vi "Test Executive.vi"() -> ()   [LabVIEW 2020]
uses:
  Library - Test Executive.llb/Test Executive - Globals.vi
  Library - Test Executive.llb/Test Executive.lvlib
panel:
  in  "Tab Control":T1(tab)
  in  "Serial Number":string
  out "Sequence":string
  out "Report Text":string
  in  "Operator":string
  in  "Save Report":bool
  in  "Clear Report Text":bool
  out "Sequence Name":string="None"
  in  "Abort Button":bool
  in  "Sequence Run":bool
  in  "Sequence Load":bool
  in  "Results Analyser":bool
  in  "Power Down":bool
  in  "Power Up":bool
  in  "Test":u16(ring) items=["1 Current Consumption", "2 Firmware Revision", "3 Indicators", "4 Gain", "5 Sensitivity"]
  in  "Check Test Equipment":bool
  out "errors":errorcluster
  in  "Power Down":bool
  in  "Power Up":bool
  in  "Reset All":bool
  in  "Run Single Test":bool
  out "Help Text":string="This is some help text\n"
  out "Abort":bool
  out "Error":bool
  out "Running":bool
  in  "Quit":bool
  # "Sequence"
  # "Progress"
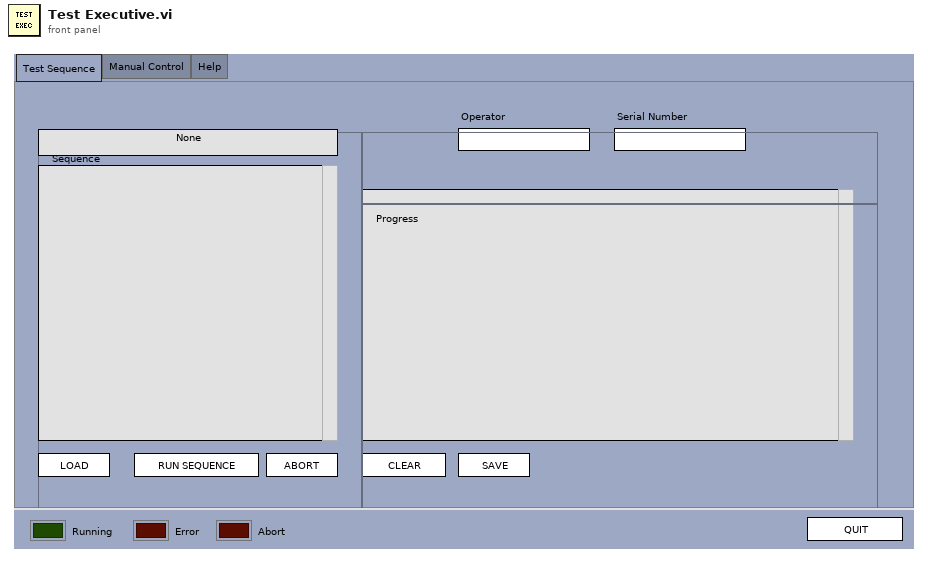
[diagram p1: front panel]
types:
  T1 = enum32{"Test Sequence", "Manual Control", "Help"}
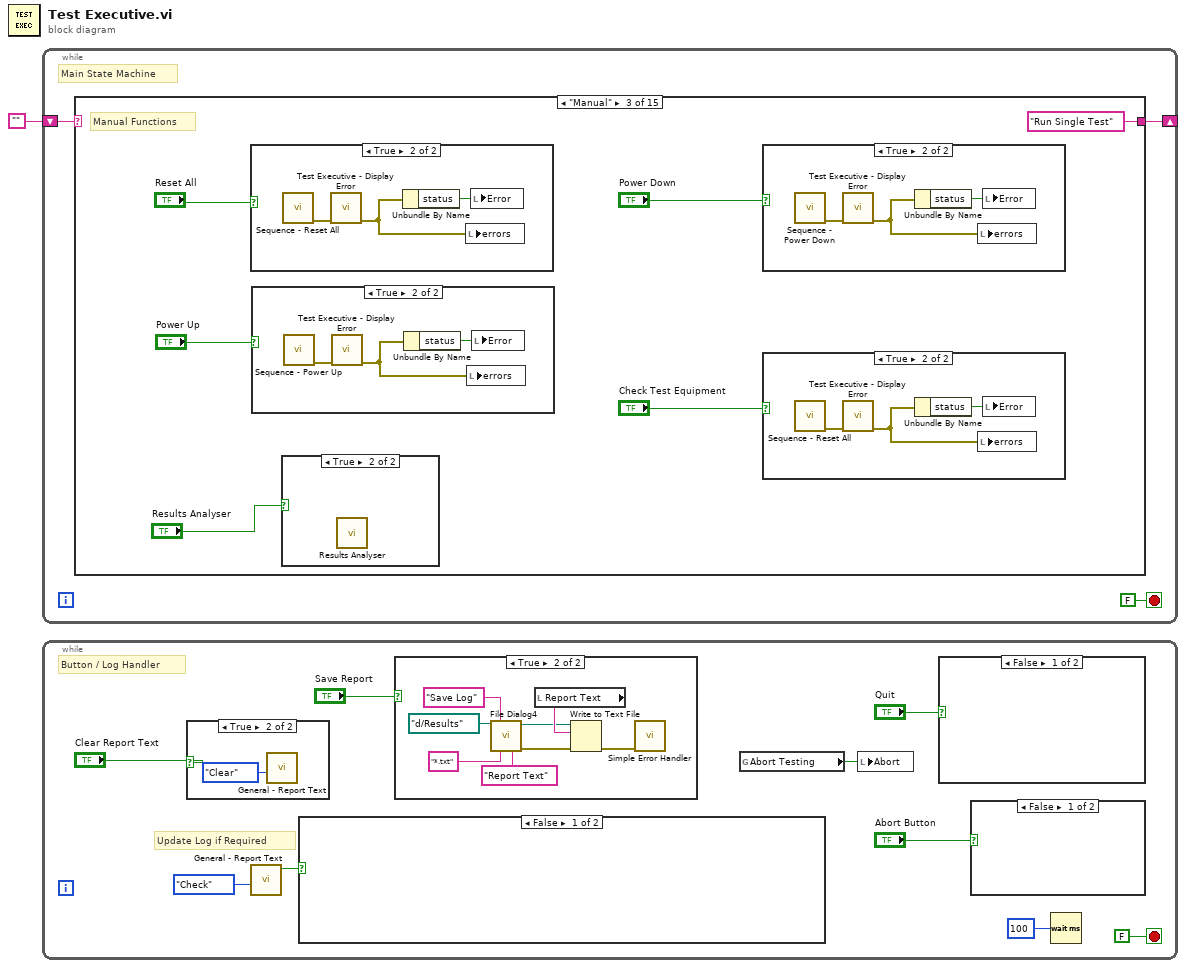
[diagram p0: block diagram]
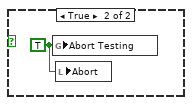
[diagram p2: hidden frame]
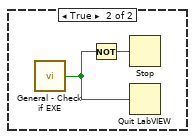
[diagram p4: hidden frame]
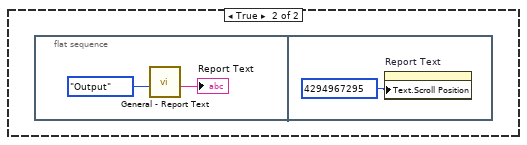
[diagram p5: hidden frame]
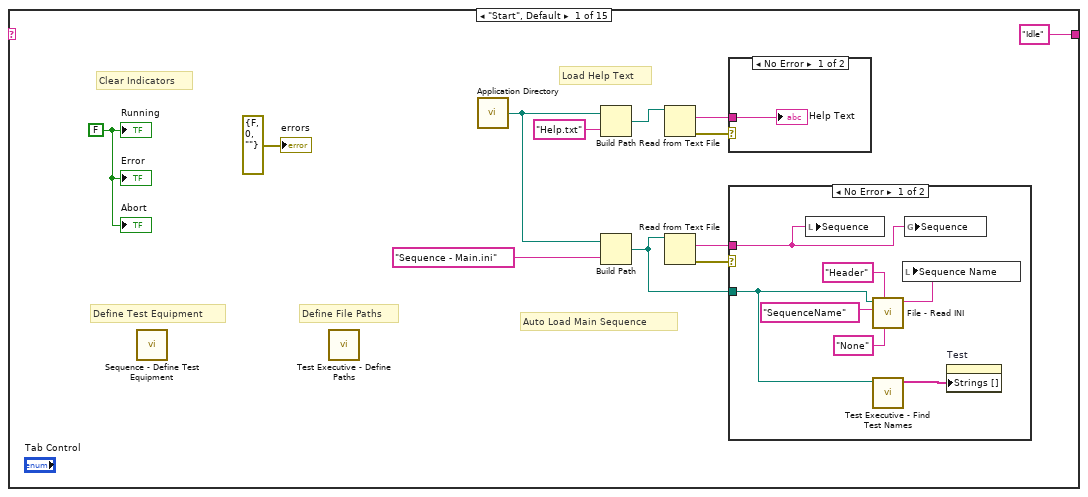
[diagram p7: hidden frame]
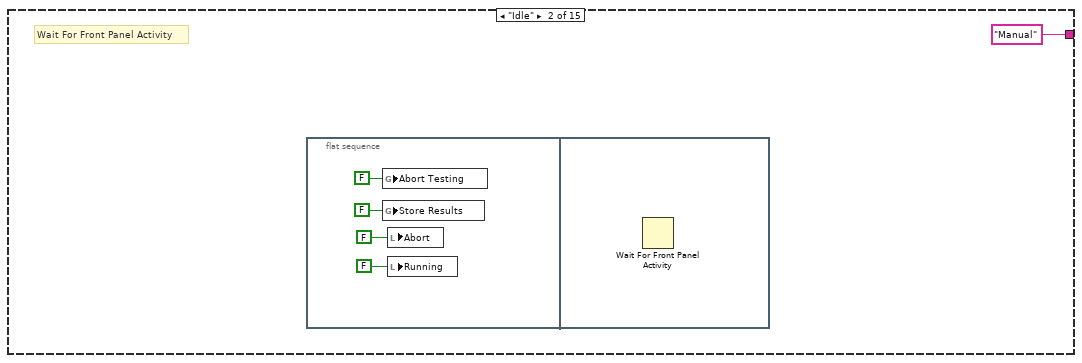
[diagram p10: hidden frame]
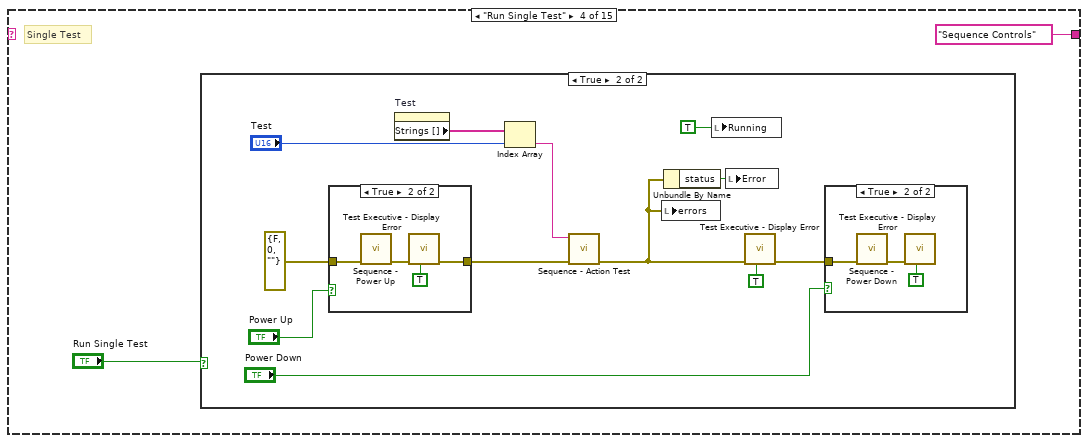
[diagram p16: hidden frame]
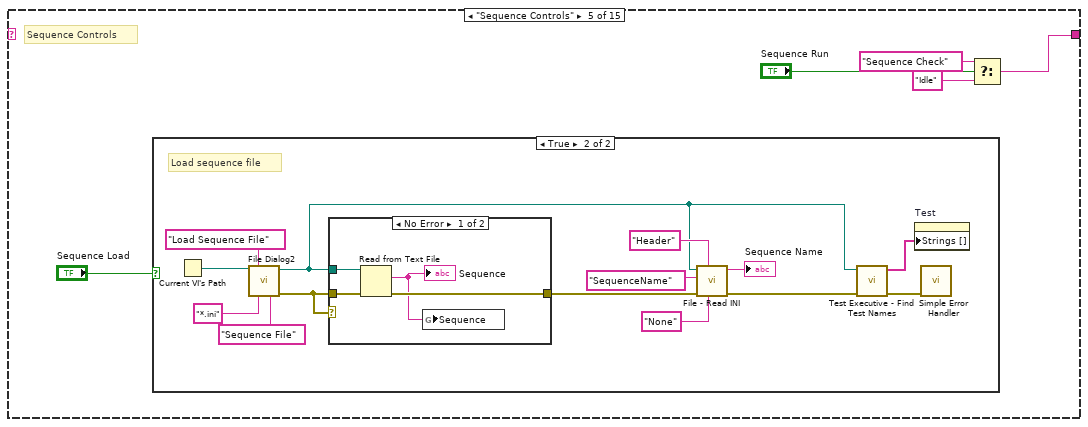
[diagram p20: hidden frame]
diagram:
  n1 = while {
    shift-right: [w2] -> _
    shift-left: "" -> [w3]
    stop <- FALSE stop-if-true
    # "Main State Machine"
    n2 = case shown="\"Manual\"" w3 {
      tunnel: ["Idle" "Manual" "Run Single Test" ("f") "Sequence Controls" w72 w94 w102 w133 "Sequence Pre-Run" ("f") "Sequence Power Up" ("f") "Sequence Running" ("f") "Sequence Power Down" ("f") "Sequence Pass Fail" ("f") "Sequence Store Results" ("f") "Idle" ("f")] -> w2
      frame "Start", Default {
        w5 = FALSE ("Running")
        # "Auto Load Main Sequence"
        # "Load Help Text"
        # "Clear Indicators"
        # "Define File Paths"
        # "Define Test Equipment"
        n3 = call "Sequence - Define Test Equipment.vi"() -> ()  [unwired: 11 in, 1 out]
        n4 = call "Test Executive - Define Paths.vi"() -> ()  [unwired: 12 in]
        n5 = call <vilib>:"Application Directory.vi"() -> ("Application Directory"=w6:path)
        n6 = Build Path(base path=w6, name or relative path="Help.txt") -> (appended path=w13:path)
        n7 = Build Path(base path=w6, name or relative path="Sequence - Main.ini") -> (appended path=w7:path)
        n8 = Read from Text File(file (use dialog)=w13) -> (text=w12:string, error out=w11:errorcluster)  [unwired: 3 in, 2 out]
        n9 = Read from Text File(file (use dialog)=w7) -> (text=w9:string, error out=w10:errorcluster)  [unwired: 3 in, 2 out]
        n10 = case shown="No Error" w11 {
          tunnel: w12 -> [w24 _]
          frame No Error {
            "Help Text" <- w24
          }
          frame Error {
          }
        }
        n11 = case shown="No Error" w10 {
          tunnel: w9 -> [w17 _]
          tunnel: w7 -> [w19 _]
          frame No Error {
            n12 = local write "Sequence"(w17) -> ()
            n13 = call "File - Read INI.vi"("Default String"="None", "Section"="Header", "Key"="SequenceName", "configuration file path"=w19) -> ("String"=w20:string)  [unwired: 6 in, 1 out]
            n14 = call "Test Executive - Find Test Names.vi"("Configuration File Path"=w19) -> ("Test Names"=w18:string[])  [unwired: 9 in, 1 out]
            n15 = local write "Sequence Name"(w20) -> ()
            n16 = global write "Test Executive - Globals.vi" "Sequence"(w17) -> ()
            n17 = property on="Test" class="Ring (strict)"("Strings []"=w18) -> ()  [unwired: 2 in, 2 out]
          }
          frame Error {
          }
        }
        "Running" <- w5
        "Error" <- w5
        "errors" <- errorcluster {"status"=FALSE, "code"=0, "source"=""} ("errors")
        "Abort" <- w5
      }
      frame "Idle" {
        # "Wait For Front Panel Activity"
        n18 = flat-sequence {
          frame #0 {
            n19 = global write "Test Executive - Globals.vi" "Abort Testing"(FALSE ("Abort Testing")) -> ()
            n20 = global write "Test Executive - Globals.vi" "Store Results"(FALSE ("Abort Testing")) -> ()
            n21 = local write "Abort"(FALSE ("Abort")) -> ()
            n22 = local write "Running"(FALSE ("Abort")) -> ()
          }
          frame #1 {
            n23 = Wait For Front Panel Activity() -> ()  [unwired: 3 in, 1 out]
          }
        }
      }
      frame "Manual" {
        # "Manual Functions"
        n24 = case shown="True" "Reset All" {
          frame False {
          }
          frame True {
            n25 = call "Sequence - Reset All.vi"() -> ("error out"=w47:errorcluster)  [unwired: 11 in]
            n26 = call "Test Executive - Display Error.vi"("error in (no error)"=w47) -> ("error out"=w45:errorcluster)  [unwired: 10 in]
            n27 = Unbundle By Name(w45) -> ("status"=w46:bool)
            n28 = local write "errors"(w45) -> ()
            n29 = local write "Error"(w46) -> ()
          }
        }
        n30 = case shown="True" "Power Up" {
          frame False {
          }
          frame True {
            n31 = call "Sequence - Power Up.vi"() -> ("error out"=w37:errorcluster)  [unwired: 11 in]
            n32 = call "Test Executive - Display Error.vi"("error in (no error)"=w37) -> ("error out"=w36:errorcluster)  [unwired: 10 in]
            n33 = Unbundle By Name(w36) -> ("status"=w38:bool)
            n34 = local write "errors"(w36) -> ()
            n35 = local write "Error"(w38) -> ()
          }
        }
        n36 = case shown="True" "Results Analyser" {
          frame False {
          }
          frame True {
            n37 = call "Results Analyser.vi"() -> ()  [unwired: 12 in]
          }
        }
        n38 = case shown="True" "Power Down" {
          frame False {
          }
          frame True {
            n39 = call "Sequence - Power Down.vi"() -> ("error out"=w43:errorcluster)  [unwired: 11 in]
            n40 = call "Test Executive - Display Error.vi"("error in (no error)"=w43) -> ("error out"=w42:errorcluster)  [unwired: 10 in]
            n41 = Unbundle By Name(w42) -> ("status"=w44:bool)
            n42 = local write "errors"(w42) -> ()
            n43 = local write "Error"(w44) -> ()
          }
        }
        n44 = case shown="True" "Check Test Equipment" {
          frame False {
          }
          frame True {
            n45 = call "Sequence - Reset All.vi"() -> ("error out"=w40:errorcluster)  [unwired: 11 in]
            n46 = call "Test Executive - Display Error.vi"("error in (no error)"=w40) -> ("error out"=w39:errorcluster)  [unwired: 10 in]
            n47 = Unbundle By Name(w39) -> ("status"=w41:bool)
            n48 = local write "errors"(w39) -> ()
            n49 = local write "Error"(w41) -> ()
          }
        }
      }
      frame "Run Single Test" {
        # "Single Test"
        n50 = case shown="True" "Run Single Test" {
          frame False {
          }
          frame True {
            n51 = case shown="True" "Power Up" {
              tunnel: errorcluster {"status"=FALSE, "code"=0, "source"=""} ("error in (no error)") -> [w65 w69]
              tunnel: [w65 w68] -> w58
              frame False {
              }
              frame True {
                n52 = call "Sequence - Power Up.vi"("error in (no error)"=w69) -> ("error out"=w67:errorcluster)  [unwired: 10 in]
                n53 = call "Test Executive - Display Error.vi"("Clear Error"=TRUE, "error in (no error)"=w67) -> ("error out"=w68:errorcluster)  [unwired: 9 in]
              }
            }
            n54 = property on="Test" class="Ring (strict)"() -> ("Strings []"=w55:string[])  [unwired: 2 in, 2 out]
            n55 = Index Array(array=w55, index="Test") -> (element=w54:string)
            n56 = call "Sequence - Action Test.vi"("error in (no error)"=w58, "Test"=w54) -> ("error out"=w50:errorcluster)  [unwired: 9 in]
            n57 = local write "errors"(w50) -> ()
            n58 = Unbundle By Name(w50) -> ("status"=w57:bool)
            n59 = local write "Running"(TRUE ("Running")) -> ()
            n60 = local write "Error"(w57) -> ()
            n61 = call "Test Executive - Display Error.vi"("Clear Error"=TRUE, "error in (no error)"=w50) -> ("error out"=w51:errorcluster)  [unwired: 9 in]
            n62 = case shown="True" "Power Down" {
              tunnel: w51 -> [_ w64]
              frame False {
              }
              frame True {
                n63 = call "Sequence - Power Down.vi"("error in (no error)"=w64) -> ("error out"=w63:errorcluster)  [unwired: 10 in]
                n64 = call "Test Executive - Display Error.vi"("Clear Error"=TRUE, "error in (no error)"=w63) -> ()  [unwired: 9 in, 1 out]
              }
            }
          }
        }
      }
      frame "Sequence Controls" {
        # "Sequence Controls"
        n65 = case shown="True" "Sequence Load" {
          frame False {
          }
          frame True {
            # "Load sequence file"
            n66 = Current VI's Path() -> (path=w86:path)
            n67 = call "File Dialog2"("start path"=w86, "prompt"="Load Sequence File", "pattern (all files)"="*.ini", "pattern label"="Sequence File") -> ("selected path"=w78:path, "error out"=w84:errorcluster)  [unwired: 8 in, 2 out]
            n68 = case shown="No Error" w84 {
              tunnel: w84 -> [w92 w93]
              tunnel: w78 -> [w91 _]
              tunnel: [w90 w93] -> w80
              frame No Error {
                n69 = Read from Text File(file (use dialog)=w91, error in=w92) -> (text=w89:string, error out=w90:errorcluster)  [unwired: 2 in, 2 out]
                "Sequence" <- w89
                n70 = global write "Test Executive - Globals.vi" "Sequence"(w89) -> ()
              }
              frame Error {
              }
            }
            n71 = call "File - Read INI.vi"("Default String"="None", "Section"="Header", "error in (no error)"=w80, "Key"="SequenceName", "configuration file path"=w78) -> ("error out"=w77:errorcluster, "String"=→"Sequence Name":string)  [unwired: 5 in]
            n72 = call "Test Executive - Find Test Names.vi"("error in (no error)"=w77, "Configuration File Path"=w78) -> ("error out"=w76:errorcluster, "Test Names"=w75:string[])  [unwired: 8 in]
            n73 = property on="Test" class="Ring (strict)"("Strings []"=w75) -> ()  [unwired: 2 in, 2 out]
            n74 = call <vilib>:"Simple Error Handler.vi"("error in (no error)"=w76) -> ()  [unwired: 4 in, 5 out]
          }
        }
        n75 = Select(t="Sequence Check", s="Sequence Run", f="Idle") -> (s? t:f=w72:string)
      }
      frame "Sequence Check" {
        # "Check Sequence Name"
        # "Sequence Check"
        n76 = local read "Sequence Name"() -> (w96:string)
        n77 = Equal?(x=w96, y="None") -> (x = y?=w98:bool)
        n78 = case shown="True" w98 {
          tunnel: "Sequence Start" -> [w99 _]
          tunnel: [w99 "Idle"] -> w94
          frame False {
          }
          frame True {
            n79 = call "Dialog Box - One Button.vi"("Text"="ERROR: Sequence name is set to \"None\".") -> ()  [unwired: 10 in, 1 out]
          }
        }
      }
      frame "Sequence Start" {
        # "Enter Serial Number"
        # "Enter Operator Name"
        # "Start of Sequence"
        # "Configure Results Storage"
        n80 = local read "Operator"() -> (w118:string)
        n81 = call <vilib>:"Dflt Data Dir.vi"() -> ("App:Default Data Directory"=w106:path)
        n82 = call "Dialog Box - Text Input.vi"("Value In"=w118, "Text"="Please enter your name") -> ("error out"=w121:errorcluster, "Value Out"=w111:string)  [unwired: 8 in]
        n83 = Build Path(base path=w106, name or relative path="Results") -> (appended path=w108:path)
        n84 = call "General - Check if Mac.vi"() -> ("Mac"=w109:bool)  [unwired: 2 in]
        n85 = Path To String(path=w108) -> (string=w107:string)
        n86 = local write "Operator"(w111) -> ()
        n87 = global write "Test Executive - Globals.vi" "Operator Name"(w111) -> ()
        n88 = case shown="True" w109 {
          tunnel: [w127 w131] -> w114
          tunnel: w107 -> [w125 w129]
          frame True {
            n89 = call "Test Executive - Sequence File Value.vi"("Default String"=w125, "Section (Current Test)"="results" ("Section"), "Key"="directorymac") -> ("String"=w127:string)  [unwired: 5 in, 3 out]
          }
          frame False {
            n90 = call "Test Executive - Sequence File Value.vi"("Default String"=w129, "Section (Current Test)"="results" ("Section"), "Key"="directorywin") -> ("String"=w131:string)  [unwired: 5 in, 3 out]
          }
        }
        n91 = local read "Serial Number"() -> (w119:string)
        n92 = String To Path(string=w114) -> (path=w112:path)
        n93 = global write "Test Executive - Globals.vi" "Results Directory"(w112) -> ()
        n94 = call "Results Storage - Setup.vi"("Rename Files on Close"=TRUE, "Results Directory"=w112) -> ()  [unwired: 9 in, 1 out]
        n95 = call "Dialog Box - Text Input.vi"("error in (no error)"=w121, "Value In"=w119, "Text"="Please enter serial number") -> ("Value Out"=w104:string)  [unwired: 7 in, 1 out]
        n96 = Empty String/Path?(string/path=w104) -> (empty?=w103:bool)
        n97 = local write "Serial Number"(w104) -> ()
        n98 = global write "Test Executive - Globals.vi" "Serial Number"(w104) -> ()
        n99 = case shown="False" w103 {
          tunnel: ["Sequence Check Equipment" ("f") "Idle" ("f")] -> w102
          frame False {
          }
          frame True {
            n100 = call "Dialog Box - One Button.vi"("Text"="ERROR: Serial number cannot be blank.") -> ()  [unwired: 10 in, 1 out]
          }
        }
        n101 = global write "Test Executive - Globals.vi" "Abort Testing"(FALSE ("Abort Testing")) -> ()
        n102 = global write "Test Executive - Globals.vi" "Unit Passed"(FALSE ("Pass")) -> ()
        n103 = call "General - Report Text.vi"("Mode (Add)"=enum16{"Add", "Output", "Clear", "Check"}."Clear") -> ()  [unwired: 8 in, 3 out]
      }
      frame "Sequence Check Equipment" {
        # "Check Test Equipment"
        # "Check Test Equipment"
        n104 = call "Sequence - Check Test Equipment.vi"() -> ("error out"=w136:errorcluster, "PASS"=w137:bool)  [unwired: 10 in]
        n105 = Not(x=w137) -> (.not. x?=w135:bool)
        n106 = case shown="True" w135 {
          tunnel: "Sequence Asset" -> [w138 _]
          tunnel: [w138 "Idle"] -> w133
          tunnel: w136 -> [_ _]
          frame False {
          }
          frame True {
            n107 = call "Dialog Box - One Button.vi"("Text"="ERROR: Test equipment check failed.") -> ()  [unwired: 10 in, 1 out]
          }
        }
      }
      frame "Sequence Asset" {
        # "Test Equipment is Defined is \"Sequence - Define Test Equipment.vi\""
        # "Enter Equipment Asset Numbers"
        n108 = global read "Test Executive - Globals.vi" "Asset Number Recording"() -> (w141:bool)
        n109 = case shown="True" w141 {
          frame False {
          }
          frame True {
            n110 = call "Test Equipment - Asset Numbers.vi"("Mode"=enum16{"Edit", "Define", "Load", "Save", "CSV"}."Load") -> ("error out"=w143:errorcluster)  [unwired: 9 in, 1 out]
            n111 = call "Test Equipment - Asset Numbers.vi"("error in (no error)"=w143, "Mode"=enum16{"Edit", "Define", "Load", "Save", "CSV"}."Edit") -> ("error out"=w144:errorcluster)  [unwired: 8 in, 1 out]
            n112 = call "Test Equipment - Asset Numbers.vi"("error in (no error)"=w144, "Mode"=enum16{"Edit", "Define", "Load", "Save", "CSV"}."Save") -> ()  [unwired: 8 in, 2 out]
          }
        }
      }
      frame "Sequence Pre-Run" {
        # "Create Results File"
        # "Record Serial Number and Operator Name"
        # "Record Start Time"
        # "Start Sequence"
        n113 = call "General - Start Stop Time.vi"("Start / Stop (Start)"=enum16{"Start", "Stop"}."Start", "Initial String"="Sequence Started") -> ("String with Time / Date"=w162:string)  [unwired: 8 in, 1 out]
        n114 = local write "Running"(TRUE ("Test Running")) -> ()
        n115 = call "General - Report Text.vi"("Mode (Add)"=enum16{"Add", "Output", "Clear", "Check"}."Add", "Text In"=w162) -> ("error out"=w153:errorcluster)  [unwired: 7 in, 2 out]
        n116 = Concatenate Strings("Serial Number: " ("string"), "Serial Number") -> (w158:string)
        n117 = call "General - Report Text.vi"("error in (no error)"=w153, "Mode (Add)"=enum16{"Add", "Output", "Clear", "Check"}."Add", "Text In"=w158) -> ("error out"=w152:errorcluster)  [unwired: 6 in, 2 out]
        n118 = global write "Test Executive - Globals.vi" "Store Results"(TRUE ("Store Results")) -> ()
        n119 = Concatenate Strings("Operator Name: " ("string"), "Operator") -> (w155:string)
        n120 = call "Results Storage - Create Results File.vi"("Operator Name"="Operator", "Serial Number"="Serial Number") -> ()  [unwired: 9 in, 1 out]
        n121 = call "General - Report Text.vi"("error in (no error)"=w152, "Mode (Add)"=enum16{"Add", "Output", "Clear", "Check"}."Add", "Text In"=w155) -> ()  [unwired: 6 in, 3 out]
      }
      frame "Sequence Power Up" {
        # "Reset all Test Equipment then Power Up Unit Under Test"
        # "Sequence Power Up"
        n122 = call "Sequence - Reset All.vi"() -> ("error out"=w169:errorcluster)  [unwired: 11 in]
        n123 = call "Test Executive - Display Error.vi"("Clear Error"=TRUE, "error in (no error)"=w169) -> ("error out"=w168:errorcluster)  [unwired: 9 in]
        n124 = call "Sequence - Power Up.vi"("error in (no error)"=w168) -> ("error out"=w167:errorcluster)  [unwired: 10 in]
        n125 = call "Test Executive - Display Error.vi"("Clear Error"=TRUE, "error in (no error)"=w167) -> ()  [unwired: 9 in, 1 out]
      }
      frame "Sequence Running" {
        # "Run Sequence"
        n126 = property on="Test" class="Ring (strict)"() -> ("Strings []"=w171:string[])  [unwired: 2 in, 2 out]
        n127 = for {
          tunnel: w171 -> [w174] mode=indexing
          stop <- w175 stop-if-true
          # "Step Through Each Test"
          n128 = call "Sequence - Action Test.vi"("Test"=w174) -> ("error out"=w173:errorcluster)  [unwired: 10 in]
          n129 = stacked-sequence {
            tunnel: [w178] -> w175
            tunnel: w173 -> [w177]
            frame #0 {
              n130 = call "Test Executive - Display Error.vi"("error in (no error)"=w177) -> ("error out"=w176:errorcluster)  [unwired: 10 in]
              n131 = global read "Test Executive - Globals.vi" "Abort Testing"() -> (w178:bool)
              n132 = Unbundle By Name(w176) -> ("status"=w179:bool)
              n133 = local write "Error"(w179) -> ()
              n134 = local write "errors"(w176) -> ()
            }
          }
        }
      }
      frame "Sequence Power Down" {
        # "Power Down Unit Under Test then Reset all Test Equipment"
        # "Sequence Power Down"
        n135 = call "Sequence - Power Down.vi"() -> ("error out"=w180:errorcluster)  [unwired: 11 in]
        n136 = call "Test Executive - Display Error.vi"("Clear Error"=TRUE, "error in (no error)"=w180) -> ("error out"=w181:errorcluster)  [unwired: 9 in]
        n137 = call "Sequence - Reset All.vi"("error in (no error)"=w181) -> ("error out"=w182:errorcluster)  [unwired: 10 in]
        n138 = call "Test Executive - Display Error.vi"("Clear Error"=TRUE, "error in (no error)"=w182) -> ()  [unwired: 9 in, 1 out]
      }
      frame "Sequence Pass Fail" {
        # "Add Stop Time"
        # "Sequence Pass / Fail"
        # "Display Banner"
        # "Pass / Fail ??"
        n139 = call "General - Report Text.vi"("Mode (Add)"=enum16{"Add", "Output", "Clear", "Check"}."Output") -> ("Report Text Out"=w195:string)  [unwired: 8 in, 2 out]
        n140 = Search/Split String(string=w195, search string/char (-)="ERROR") -> (offset of match=w215:i32)  [unwired: 1 in, 2 out]
        n141 = Search/Split String(string=w195, search string/char (-)="FAIL") -> (offset of match=w209:i32)  [unwired: 1 in, 2 out]
        n142 = Search/Split String(string=w195, search string/char (-)="PASS") -> (offset of match=w196:i32)  [unwired: 1 in, 2 out]
        n143 = Greater Than 0?(x=w215) -> (x > 0?=w216:bool)
        n144 = Greater Than 0?(x=w209) -> (x > 0?=w210:bool)
        n145 = Greater Than 0?(x=w196) -> (x > 0?=w193:bool)
        n146 = Select(t="UNIT PASSED", s=w193, f="UNIT FAILED") -> (s? t:f=w192:string)
        n147 = Select(t="UNIT FAILED", s=w210, f=w192) -> (s? t:f=w217:string)
        n148 = Select(t="UNIT FAILED (ERRORS)", s=w216, f=w217) -> (s? t:f=w190:string)
        n149 = global read "Test Executive - Globals.vi" "Abort Testing"() -> (w187:bool)
        n150 = Select(t="TESTING ABORTED", s=w187, f=w190) -> (s? t:f=w188:string)
        n151 = Select(t="Sequence Aborted", s=w187, f="Sequence Completed" ("Initial String")) -> (s? t:f=w204:string)
        n152 = call "General - Report Text.vi"("Mode (Add)"=enum16{"Add", "Output", "Clear", "Check"}."Add", "Text In"=w188) -> ("error out"=w200:errorcluster)  [unwired: 7 in, 2 out]
        n153 = call "General - Start Stop Time.vi"("Start / Stop (Start)"=enum16{"Start", "Stop"}."Stop", "Initial String"=w204) -> ("String with Time / Date"=w202:string)  [unwired: 8 in, 1 out]
        n154 = Equal?(x="UNIT PASSED", y=w188) -> (x = y?=w186:bool)
        n155 = global write "Test Executive - Globals.vi" "Unit Passed"(w186) -> ()
        n156 = call "Dialog Box - Pass Fail Banner.vi"("Pass"=w186, "Text"=w188) -> ()  [unwired: 9 in, 1 out]
        n157 = call "General - Report Text.vi"("error in (no error)"=w200, "Mode (Add)"=enum16{"Add", "Output", "Clear", "Check"}."Add", "Text In"=w202) -> ()  [unwired: 6 in, 3 out]
      }
      frame "Sequence Store Results" {
        # "Record Asset Numbers"
        # "Sequence Store Results"
        # "Close Results File"
        n158 = global read "Test Executive - Globals.vi" "Asset Number Recording"() -> (w221:bool)
        n159 = global read "Test Executive - Globals.vi" "Unit Passed"() -> (w218:bool)
        n160 = case shown="True" w221 {
          tunnel: [_ w229] -> w220
          frame False {
          }
          frame True {
            n161 = call "Test Equipment - Asset Numbers.vi"("Mode"=enum16{"Edit", "Define", "Load", "Save", "CSV"}."CSV") -> ("Output"=w230:string)  [unwired: 9 in, 1 out]
            n162 = call "Results Storage - Add Text.vi"("Add New Line (True)"=FALSE, "Text"=w230) -> ("error out"=w229:errorcluster)  [unwired: 9 in]
          }
        }
        n163 = global read "Test Executive - Globals.vi" "Abort Testing"() -> (w219:bool)
        n164 = Select(t=enum16{"auto", "passed", "failed", "aborted"}."passed" ("Result (auto)"), s=w218, f=enum16{"auto", "passed", "failed", "aborted"}."failed" ("Result (auto)")) -> (s? t:f=w223:enum16{"auto", "passed", "failed", "aborted"})
        n165 = Select(t=enum16{"auto", "passed", "failed", "aborted"}."aborted" ("Result (auto)"), s=w219, f=w223) -> (s? t:f=w222:enum16{"auto", "passed", "failed", "aborted"})
        n166 = call "Results Storage - Close Results File.vi"("error in (no error)"=w220, "Result (auto)"=w222) -> ()  [unwired: 9 in, 1 out]
      }
    }
  }
  n167 = while {
    stop <- FALSE stop-if-true
    # "Button / Log Handler"
    # "Update Log if Required"
    n168 = case shown="True" "Clear Report Text" {
      frame False {
      }
      frame True {
        n169 = call "General - Report Text.vi"("Mode (Add)"=enum16{"Add", "Output", "Clear", "Check"}."Clear") -> ()  [unwired: 8 in, 3 out]
      }
    }
    n170 = call "General - Report Text.vi"("Mode (Add)"=enum16{"Add", "Output", "Clear", "Check"}."Check") -> ("Changed Out"=w238:bool)  [unwired: 8 in, 2 out]
    n171 = case shown="False" w238 {
      frame False {
      }
      frame True {
        n172 = flat-sequence {
          frame #0 {
            n173 = call "General - Report Text.vi"("Mode (Add)"=enum16{"Add", "Output", "Clear", "Check"}."Output") -> ("Report Text Out"=→"Report Text":string)  [unwired: 8 in, 2 out]
          }
          frame #1 {
            n174 = property on="Report Text" class="Str"("Text.Scroll Position"=u32 4294967295) -> ()  [unwired: 2 in, 2 out]
          }
        }
      }
    }
    n175 = case shown="True" "Save Report" {
      frame False {
      }
      frame True {
        n176 = call "File Dialog4"("start path"=path "d:/Results", "prompt"="Save Log", "pattern (all files)"="*.txt", "pattern label"="Report Text") -> ("selected path"=w242:path, "error out"=w248:errorcluster)  [unwired: 8 in, 2 out]
        n177 = local read "Report Text"() -> (w247:string)
        n178 = Write to Text File(file (use dialog)=w242, text=w247, error in=w248) -> (error out=w249:errorcluster)  [unwired: 1 in, 2 out]
        n179 = call <vilib>:"Simple Error Handler.vi"("error in (no error)"=w249) -> ()  [unwired: 4 in, 5 out]
      }
    }
    n180 = global read "Test Executive - Globals.vi" "Abort Testing"() -> (w232:bool)
    n181 = local write "Abort"(w232) -> ()
    n182 = case shown="False" "Quit" {
      frame False {
      }
      frame True {
        n183 = call "General - Check if EXE.vi"() -> ("EXE"=w251:bool)  [unwired: 2 in]
        n184 = Not(x=w251) -> (.not. x?=w250:bool)
        n185 = Stop(stop? (T)=w250) -> ()
        n186 = Quit LabVIEW(quit? (T)=w251) -> ()
      }
    }
    n187 = case shown="False" "Abort Button" {
      frame False {
      }
      frame True {
        w241 = TRUE ("Abort Testing")
        n188 = global write "Test Executive - Globals.vi" "Abort Testing"(w241) -> ()
        n189 = local write "Abort"(w241) -> ()
      }
    }
    n190 = Wait (ms)(milliseconds to wait=u32 100) -> ()  [unwired: 1 out]
  }
